vi "TCPIP Read Hand Scanner.vi"(9 "Mode":enum16{"Init", "Read", "Close"}(ring)=enum."Close", 10 "remote port or service name":u16=9004, 11 "address":string="172.17.53.83") -> (3 "String":string)   [LabVIEW 2018]
panel:
  out "error out":errorcluster
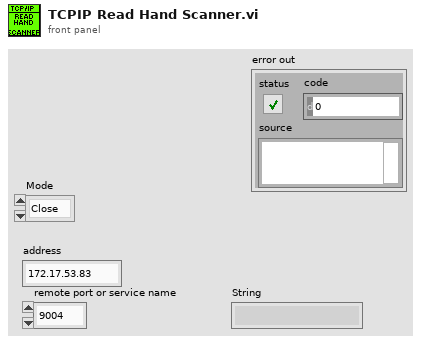
[diagram p1: front panel]
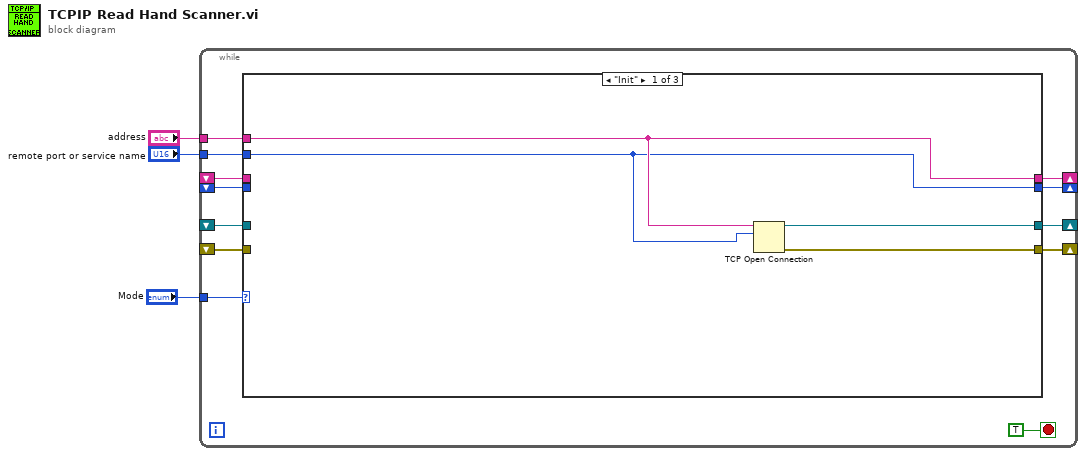
[diagram p0: block diagram]
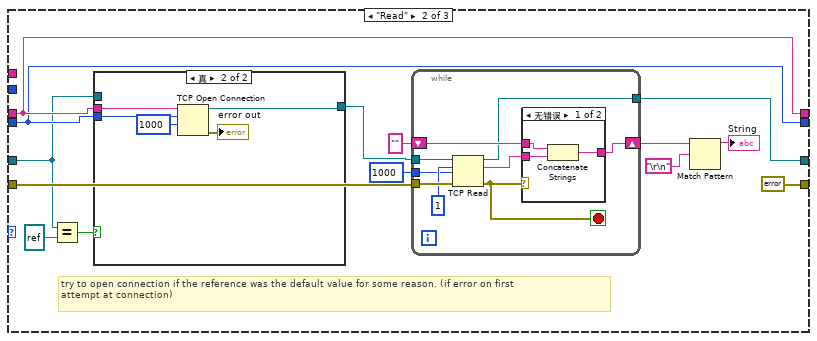
[diagram p2: hidden frame]
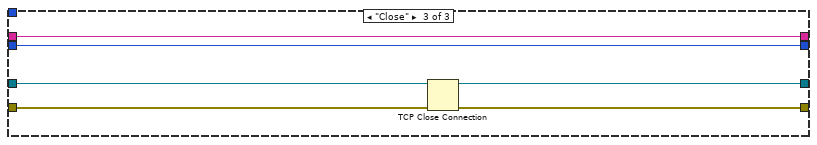
[diagram p5: hidden frame]
diagram:
  n1 = while {
    tunnel: "Mode" -> [w14]
    shift-right: [w13] -> _
    shift-left: _ -> [w11]
    shift-right: [w12] -> _
    shift-left: _ -> [w10]
    shift-right: [w7] -> _
    shift-left: _ -> [w4]
    shift-right: [w9] -> _
    shift-left: _ -> [w5]
    tunnel: "address" -> [w8]
    tunnel: "remote port or service name" -> [w6]
    stop <- TRUE stop-if-true
    n2 = case shown="\"Init\"" w14 {
      tunnel: [w19 w30 w55] -> w13
      tunnel: [w18 errorcluster {"status"=FALSE, "code"=0, "source"=""} ("error out") w56] -> w12
      tunnel: w11 -> [_ w21 w58]
      tunnel: w10 -> [_ w31 w57]
      tunnel: [w17 w23 w54] -> w9
      tunnel: w8 -> [w17 _ _]
      tunnel: [w16 w22 w53] -> w7
      tunnel: w6 -> [w16 _ _]
      tunnel: w5 -> [_ w23 w54]
      tunnel: w4 -> [_ w22 w53]
      frame "Init" {
        n3 = TCP Open Connection(address=w17, remote port or service name=w16) -> (connection ID=w19:refnum<k5>, error out=w18:errorcluster)  [unwired: 3 in]
      }
      frame "Read" {
        # "try to open connection if the reference was the default value for some reason. (if error on first\nattempt at connection)"
        n4 = Equal?(x=w21, y=refnum<k5> refnum ("connection ID")) -> (x = y?=w25:bool)
        n5 = case shown="真" w25 {
          tunnel: w21 -> [w34 _]
          tunnel: [w34 w36] -> w20
          tunnel: w23 -> [_ w39]
          tunnel: w22 -> [_ w38]
          frame False {
          }
          frame True {
            n6 = TCP Open Connection(address=w39, remote port or service name=w38, timeout ms (60000)=1000) -> (connection ID=w36:refnum<k5>, error out=→"error out":errorcluster)  [unwired: 2 in]
          }
        }
        n7 = while {
          tunnel: w20 -> [w48]
          tunnel: w31 -> [w47]
          shift-right: [w44] -> w27
          shift-left: "" -> [w43]
          tunnel: 1000 ("timeout ms (25000)") -> [w42]
          tunnel: [w40] -> w30
          stop <- w41 stop-if-true
          n8 = TCP Read(connection ID=w48, bytes to read=1, error in (no error)=w47, 9:w42) -> (connection ID out=w40:refnum<k5>, data out=w45:string, error out=w41:errorcluster)  [unwired: 1 in]
          n9 = case shown="无错误" w41 {
            tunnel: w45 -> [w50 _]
            tunnel: [w49 w52] -> w44
            tunnel: w43 -> [w51 w52]
            frame No Error {
              n10 = Concatenate Strings(w51, w50) -> (w49:string)
            }
            frame Error {
            }
          }
        }
        n11 = Match Pattern(string=w27, regular expression="\r\n") -> (before substring=→"String":string)  [unwired: 1 in, 3 out]
      }
      frame "Close" {
        n12 = TCP Close Connection(connection ID=w58, error in (no error)=w57) -> (connection ID out=w55:refnum<k5>, error out=w56:errorcluster)  [unwired: 1 in]
      }
    }
  }
